vi "is input.vi"(8 "error in (no error)":errorcluster, 11 "Item Ref in":T1 format="%.0x") -> (0 "error out":errorcluster, 2 "input?":bool, 3 "Channel Ref out":T1 format="%.0x")   [LabVIEW 2021, in "Modbus Master System Explorer.lvlib"]
uses:
  Modbus Master System Explorer.lvlib
  <vilib>/NI VeriStand/Custom Device API/Custom Device Item Ref.ctl
  <vilib>/NI VeriStand/Custom Device API/Custom Device Channel Type.ctl
  <vilib>/NI VeriStand/Custom Device API/Custom Device API.lvlib
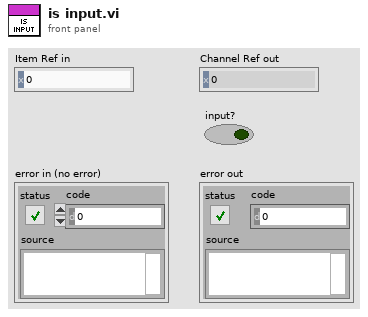
[diagram p1: front panel]
types:
  T1 = typedef "Custom Device API.lvlib/Custom Device Item Ref.ctl" = u64
  T2 = typedef "Custom Device API.lvlib/Custom Device Channel Type.ctl" = enum16{"Input", "Output"}
  T3 = typedef "Custom Device API.lvlib/Custom Device Channel.ctl" = cluster{"Type":T2, "Units":string, "Default Value":dbl, "Faultable":bool, "Scalable":bool}
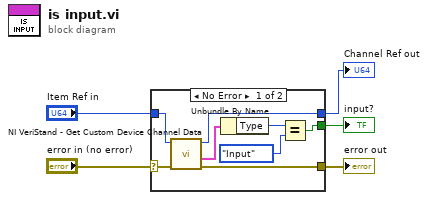
[diagram p0: block diagram]
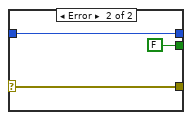
[diagram p2: hidden frame]
diagram:
  n1 = case shown="No Error" "error in (no error)" {
    selector: "error in (no error)" -> [w12 w15]
    tunnel: [w13 w15] -> w5
    tunnel: [w11 FALSE] -> w3
    tunnel: [w7 w16] -> w2
    tunnel: "Item Ref in" -> [w6 w16]
    frame No Error {
      n2 = call <vilib>:"NI VeriStand - Get Custom Device Channel Data.vi"("error in (no error)"=w12, "Channel Ref in"=w6) -> ("error out"=w13:errorcluster, "Channel"=w8:T3, "Channel Ref out"=w7:T1)  [unwired: 4 in, 3 out]
      n3 = Unbundle By Name(w8) -> ("Type"=w9:T2)
      n4 = Equal?(x=w9, y=Custom_Device_Channel_Type."Input") -> (x = y?=w11:bool)
    }
    frame Error {
    }
  }
  "error out" <- w5
  "input?" <- w3
  "Channel Ref out" <- w2
